vi "CREATE ARCHIVE ITEM SQL QUERY.vi"(0 "What to Search":string, 5 "Search Column Name":string, 7 "Sorting Column Name":string, 9 "Column to Search In":u16, 12 "Date Range":u16(ring) items=["Greater Than", "Less Than", "Between"], 13 "Dates Less Than":string="8/1/2023", 14 "Dates Greater Than":string="8/1/2023") -> (4 "SQL QUERY":string)   [LabVIEW 2019]
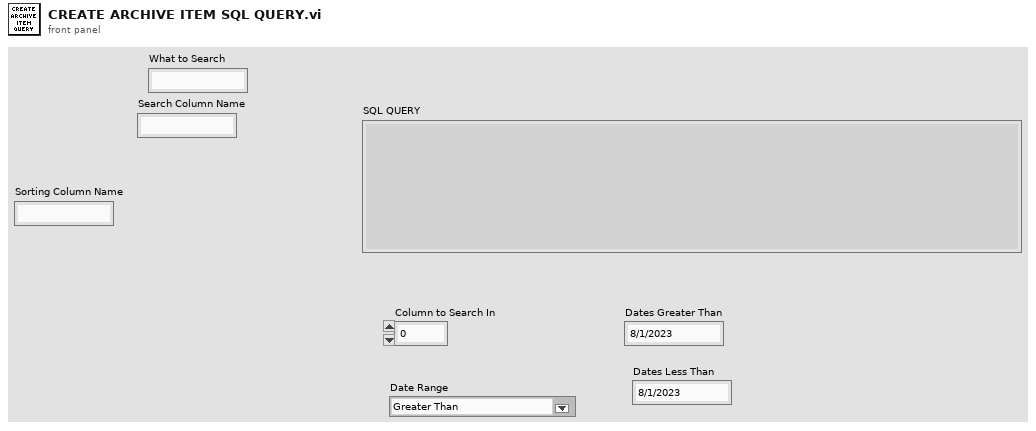
[diagram p1: front panel]
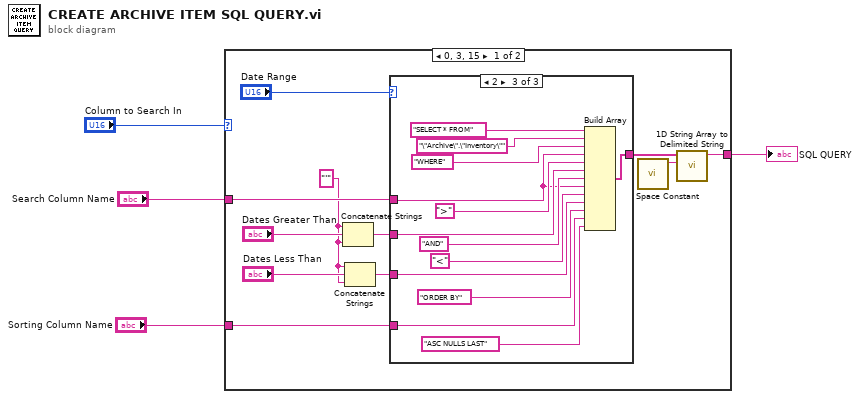
[diagram p0: block diagram]
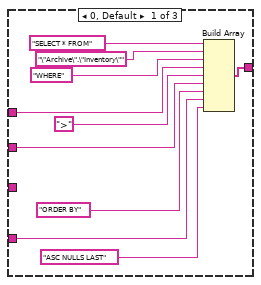
[diagram p2: hidden frame]
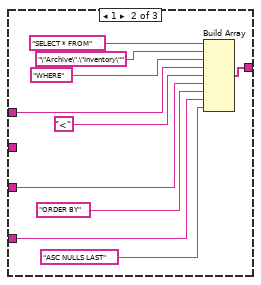
[diagram p3: hidden frame]
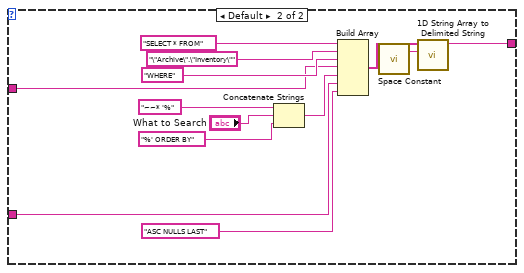
[diagram p4: hidden frame]
diagram:
  n1 = case shown="0, 3, 15" "Column to Search In" {
    tunnel: [w13 w60] -> w4
    tunnel: "Sorting Column Name" -> [w10 w50]
    tunnel: "Search Column Name" -> [w12 w49]
    frame 0, 3, 15 {
      w5 = "'"
      n2 = Concatenate Strings(w5, "Dates Greater Than", w5) -> (w9:string)
      n3 = Concatenate Strings(w5, "Dates Less Than", w5) -> (w8:string)
      n4 = case shown="2" "Date Range" {
        tunnel: w12 -> [w22 w32 w41]
        tunnel: w9 -> [w20 _ w43]
        tunnel: [w19 w30 w44] -> w11
        tunnel: w10 -> [w17 w28 w37]
        tunnel: w8 -> [_ w26 w39]
        frame 0, Default {
          n5 = Build Array("SELECT * FROM" ("string"), "\"Archive\".\"Inventory\"" ("string"), "WHERE" ("string"), w22, ">" ("string"), w20, "ORDER BY" ("string"), w17, "ASC NULLS LAST" ("string")) -> (w19:string[])
        }
        frame 1 {
          n6 = Build Array("SELECT * FROM" ("string"), "\"Archive\".\"Inventory\"" ("string"), "WHERE" ("string"), w32, "<" ("string"), w26, "ORDER BY" ("string"), w28, "ASC NULLS LAST" ("string")) -> (w30:string[])
        }
        frame 2 {
          n7 = Build Array("SELECT * FROM" ("string"), "\"Archive\".\"Inventory\"" ("string"), "WHERE" ("string"), w41, ">" ("string"), w43, "AND" ("string"), w41, "<" ("string"), w39, "ORDER BY" ("string"), w37, "ASC NULLS LAST" ("string")) -> (w44:string[])
        }
      }
      n8 = call <vilib>:"Space Constant.vi"() -> ("String"=w14:string)
      n9 = call <vilib>:"1D String Array to Delimited String.vi"("delimiter"=w14, "string array"=w11) -> ("delimited string"=w13:string)  [unwired: 9 in]
    }
    frame Default {
      n10 = Concatenate Strings("~~* '%" ("string"), "What to Search", "%' ORDER BY" ("string")) -> (w52:string)
      n11 = Build Array("SELECT * FROM" ("string"), "\"Archive\".\"Inventory\"" ("string"), "WHERE" ("string"), w49, w52, w50, "ASC NULLS LAST" ("string")) -> (w58:string[])
      n12 = call <vilib>:"Space Constant.vi"() -> ("String"=w57:string)
      n13 = call <vilib>:"1D String Array to Delimited String.vi"("delimiter"=w57, "string array"=w58) -> ("delimited string"=w60:string)  [unwired: 9 in]
    }
  }
  "SQL QUERY" <- w4
